vi "Statistics.vi"(6 "Clear Channel List (empty)":string, 7 "Clear Statistics? (F:No)":bool, 8 "error in (no error)":errorcluster, 9 "Channel (0)":u16, 10 "Statistic (0:Minimum)":T1(ring), 11 "VISA Resource Name":refnum<visa-resource-name>) -> (0 "error out":errorcluster, 1 "Statistic Value":dbl format="%.2f", 2 "Time (Min/Max)":string, 3 "VISA Resource Name Out":refnum<visa-resource-name>)   [LabVIEW 2016, in "Agilent 34970.lvlib"]
doc: "This VI allows you to recall statistics data on a specified channel. You can find the Minimum, Maximum, Average, Peak-to-Peak, or Count. For Minimum and Maximum, a time stamp is also reported.\n\nAlternatively, you can clear all values from the instrument's statistics registers."
uses:
  Agilent 34970.lvlib
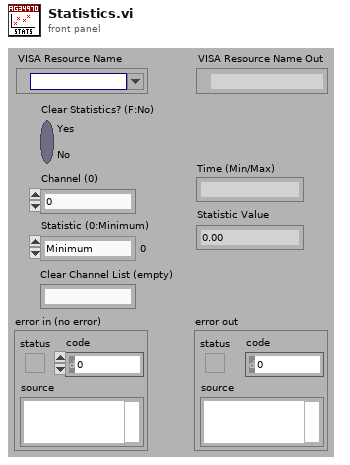
[diagram p1: front panel]
types:
  T1 = enum16{"Minimum", "Maximum", "Average", "Peak to Peak", "Count"}
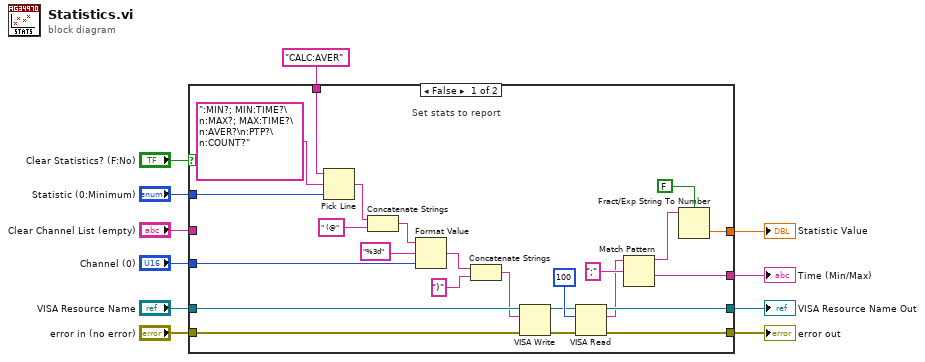
[diagram p0: block diagram]
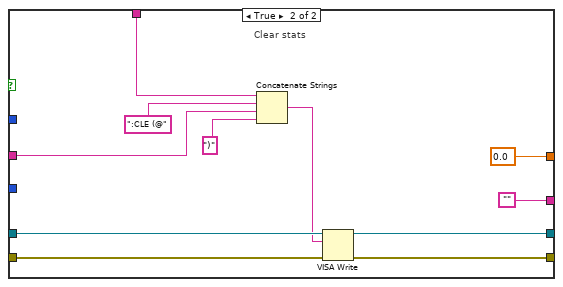
[diagram p2: hidden frame]
diagram:
  n1 = case shown="False" "Clear Statistics? (F:No)" {
    tunnel: "Statistic (0:Minimum)" -> [w32 _]
    tunnel: "Channel (0)" -> [w12 _]
    tunnel: "VISA Resource Name" -> [w27 w42]
    tunnel: "error in (no error)" -> [w26 w41]
    tunnel: [w18 w40] -> w3
    tunnel: [w16 ""] -> w8
    tunnel: [w17 w39] -> w1
    tunnel: "CALC:AVER" ("string (\"\")") -> [w22 w46]
    tunnel: "Clear Channel List (empty)" -> [_ w44]
    tunnel: [w19 0.0] -> w5
    frame False {
      # "Set stats to report"
      n2 = Pick Line(string ("")=w22, multi-line string=":MIN?; MIN:TIME?\n:MAX?; MAX:TIME?\n:AVER?\n:PTP?\n:COUNT?", line index=w32) -> (output string=w34:string)
      n3 = Concatenate Strings(w34, " (@") -> (w30:string)
      n4 = Format Value(string ("")=w30, format string="%3d", value (0)=w12) -> (output string=w28:string)
      n5 = Concatenate Strings(w28, ")") -> (w13:string)
      n6 = VISA Write(VISA resource name=w27, write buffer=w13, error in (no error)=w26) -> (VISA resource name out=w24:refnum<visa-resource-name>, error out=w23:errorcluster)  [unwired: 1 out]
      n7 = VISA Read(VISA resource name=w24, byte count=u32 100 ("byte count (0)"), error in (no error)=w23) -> (VISA resource name out=w18:refnum<visa-resource-name>, read buffer=w15:string, error out=w17:errorcluster)  [unwired: 1 out]
      n8 = Match Pattern(string=w15, regular expression=";" ("search char (-)")) -> (before substring=w20:string, after substring=w16:string)  [unwired: 1 in, 2 out]
      n9 = Fract/Exp String To Number(use system decimal point (T)=FALSE, string=w20) -> (number=w19:dbl)  [unwired: 2 in, 1 out]
    }
    frame True {
      # "Clear stats"
      n10 = Concatenate Strings(w46, ":CLE (@", w44, ")" ("Clear Channel List")) -> (w37:string)
      n11 = VISA Write(VISA resource name=w42, write buffer=w37, error in (no error)=w41) -> (VISA resource name out=w40:refnum<visa-resource-name>, error out=w39:errorcluster)  [unwired: 1 out]
    }
  }
  "Time (Min/Max)" <- w8
  "Statistic Value" <- w5
  "error out" <- w1
  "VISA Resource Name Out" <- w3
